vi "Read Incoming Bytes.vi"(8 "error in (no error)":errorcluster, 9 "timeout (1000 ms)":i32=1000, 10 "bytes to read (100)":i32=100, 11 "Connection.TCP":refnum<class "Connection.TCP.lvclass">) -> (0 "error out":errorcluster, 1 "timed out":bool, 2 "Bytes":u8[](array[numeric]) format="%08b", 3 "Connection.TCP":refnum<class "Connection.TCP.lvclass">, 4 "connected":bool)   [LabVIEW 2013, in "Connection.TCP_GOSPL.lvlib" / "Connection.TCP.lvclass"]
uses:
  Connection.TCP.lvclass
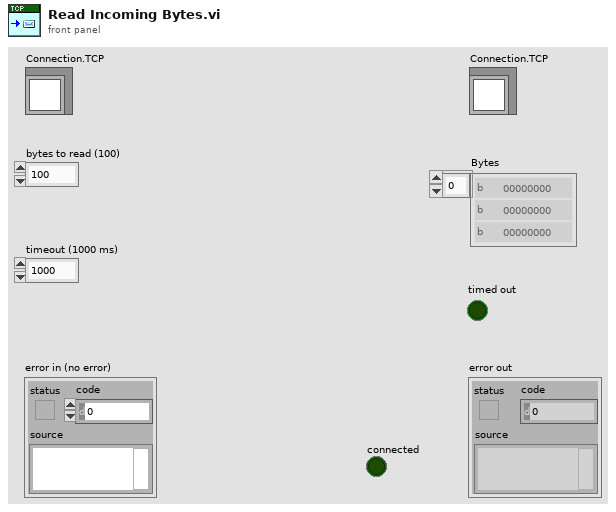
[diagram p1: front panel]
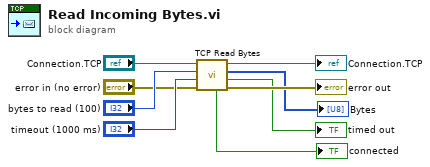
[diagram p0: block diagram]
diagram:
  n1 = call "TCP Read Bytes.vi"("error in (no error)"="error in (no error)", "timeout (1000 ms)"="timeout (1000 ms)", "bytes to read (100)"="bytes to read (100)", "Connection.TCP"="Connection.TCP") -> ("error out"=→"error out":errorcluster, "timed out"=→"timed out":bool, "Bytes"=→"Bytes":u8[], "Connection.TCP"=→"Connection.TCP":refnum<class "Connection.TCP.lvclass">, "connected"=→"connected":bool)  [unwired: 3 in]
